vi "Digital Input DAQ Engine.vi"(8 "error in":errorcluster, 10 "DAQ Engine":refnum<notifier>, 11 "Sequence Context In":refnum<k7>) -> (0 "error out":errorcluster)   [LabVIEW 2023, in "LTT_TeststandSteptypes.lvlib"]
uses:
  LTT_TeststandSteptypes.lvlib
  HardwareAbstractionLayer_LVOOP/Main/Class Ref.ctl
  HardwareAbstractionLayer_LVOOP/DMM/DMM.lvclass
  HardwareAbstractionLayer_LVOOP/Function Generator/Function Generator.lvclass
  HardwareAbstractionLayer_LVOOP/Oscilloscope/Oscilloscope.lvclass
  HardwareAbstractionLayer_LVOOP/PowerSupply/PowerSupply.lvclass
  HardwareAbstractionLayer_LVOOP/Teststand/Teststand.lvclass
  HardwareAbstractionLayer_LVOOP/Analog Output/AO/AO.lvclass
  HardwareAbstractionLayer_LVOOP/Analog Input/AI/AI.lvclass
  HardwareAbstractionLayer_LVOOP/Database/Database.lvclass
  HardwareAbstractionLayer_LVOOP/Digital Output/DO_class/DO.lvclass
  HardwareAbstractionLayer_LVOOP/Digital Input/DI_class/DI.lvclass
  HardwareAbstractionLayer_LVOOP/PWM Output/PWM Output_class/PWM Output.lvclass
  HardwareAbstractionLayer_LVOOP/PWM Input/PWM Input_class/PWM Input.lvclass
  HardwareAbstractionLayer_LVOOP/NI Switch/NISwitch_class/NISwitch.lvclass
  HardwareAbstractionLayer_LVOOP/Modbus/Modbus_class/Modbus.lvclass
  HardwareAbstractionLayer_LVOOP/CAN/CAN Lib/CAN_class/CAN.lvclass
  HardwareAbstractionLayer_LVOOP/Digital Input/NI Digital Input_class/NI Digital Input.lvclass
  D:/eDCU LTT/VT LTT Project/Source Code/HardwareAbstractionLayer_LVOOP/Digital Input/DI_class/DI.lvclass
  HardwareAbstractionLayer_LVOOP/Main/Class Options.ctl
  <vilib>/Utility/error.llb/DialogType.ctl
  HardwareAbstractionLayer_LVOOP/Main/Main.lvclass
panel:
  in  "stop":bool
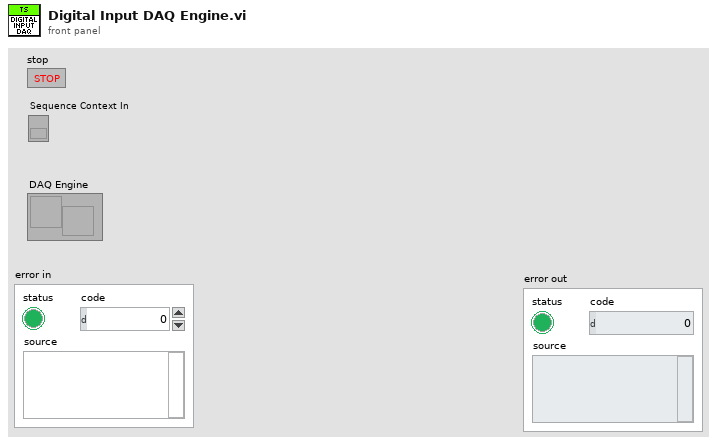
[diagram p1: front panel]
types:
  T1 = typedef "HardwareAbstractionLayer_LVOOP.lvlib/Main.lvclass/Class Ref.ctl" = cluster{"DMM":refnum<class "DMM.lvclass">, "Function Generator":refnum<class "Function Generator.lvclass">, "Oscilloscope":refnum<class "Oscilloscope.lvclass">, "PowerSupply":refnum<class "PowerSupply.lvclass">, "Teststand":refnum<class "Teststand.lvclass">, "AO":refnum<class "AO.lvclass">, "AI":refnum<class "AI.lvclass">, "Database":refnum<class "Database.lvclass">, "AO Waveform Generation":refnum<class "AO.lvclass">, "DO":refnum<class "DO.lvclass">, "DI":refnum<class "DI.lvclass">, "PWM Output":refnum<class "PWM Output.lvclass">, "PWM Input":refnum<class "PWM Input.lvclass">, "RelayOutput":refnum<class "NISwitch.lvclass">, "Modbus":refnum<class "Modbus.lvclass">, "CAN":refnum<class "CAN.lvclass">}
  T2 = typedef "HardwareAbstractionLayer_LVOOP.lvlib/Main.lvclass/Class Options.ctl" = enum16{"Init All Class", "Read All Class", "Write AI Class", "Write AO Class", "Write AO Waveform Generation", "Write DI Class", "Write DO Class", "Write PWM Input Class", "Write PWM Output Class", "Exit"}
  T3 = typedef "DialogType.ctl" = u16
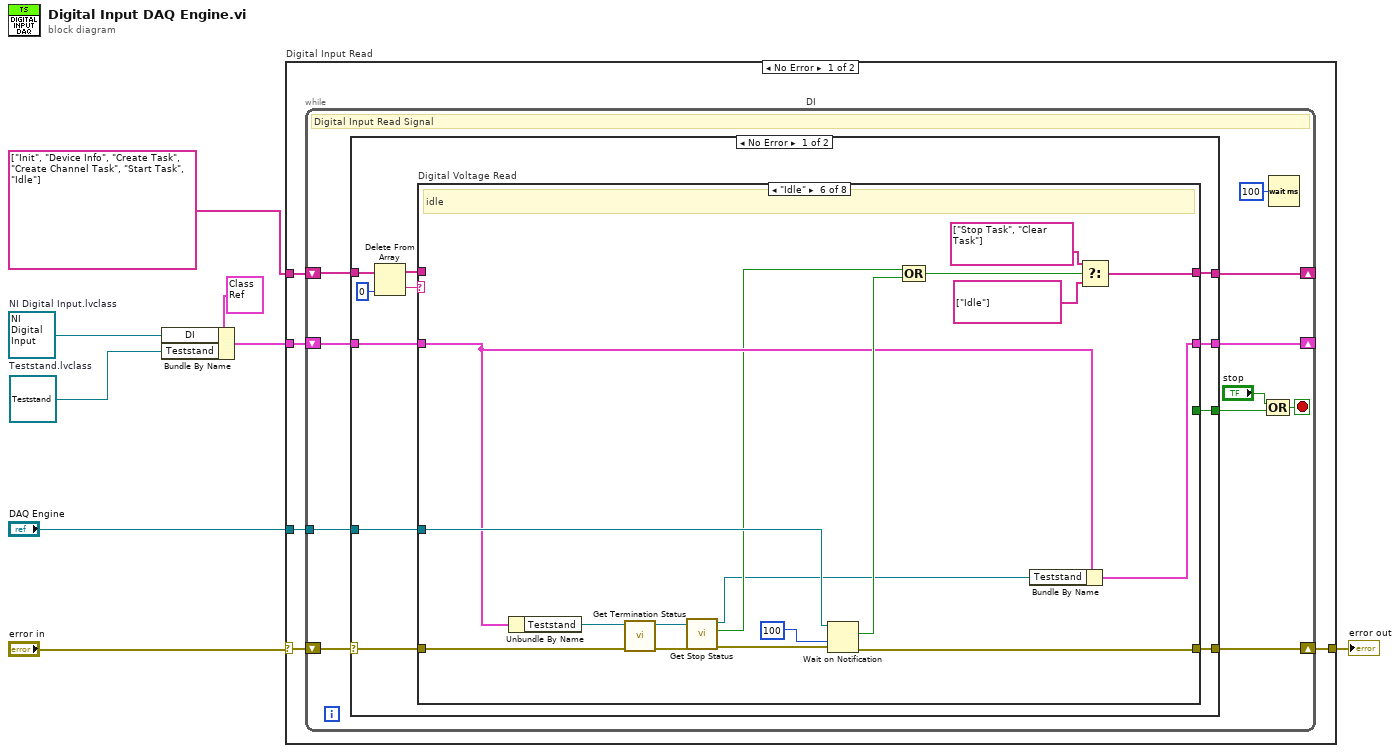
[diagram p0: block diagram]
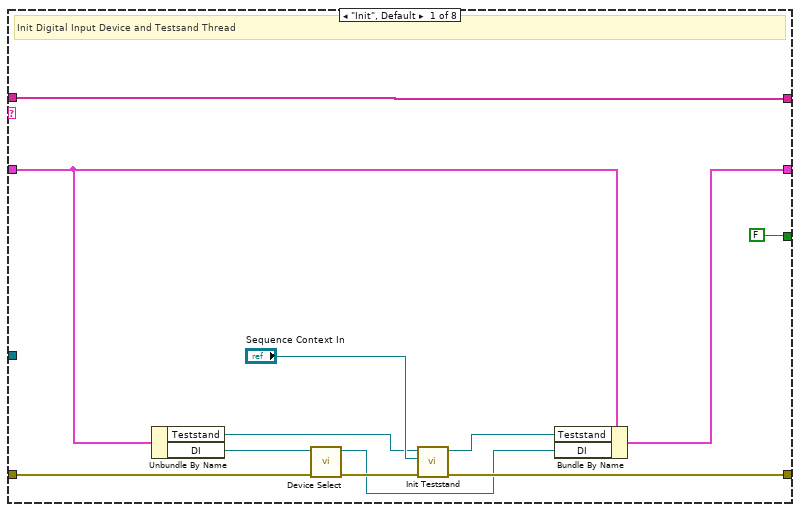
[diagram p2: hidden frame]
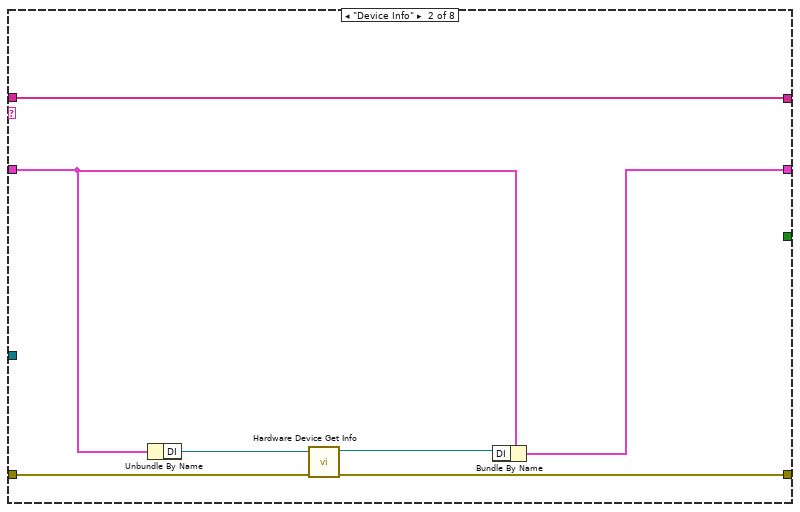
[diagram p3: hidden frame]
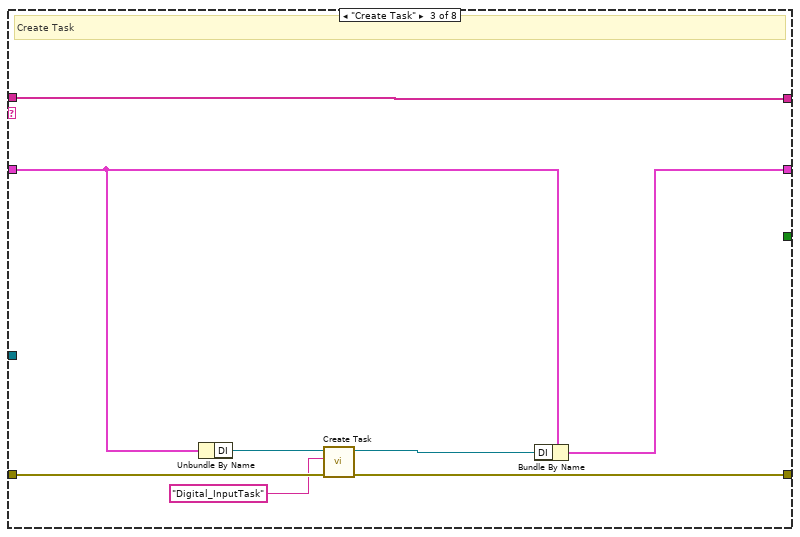
[diagram p4: hidden frame]
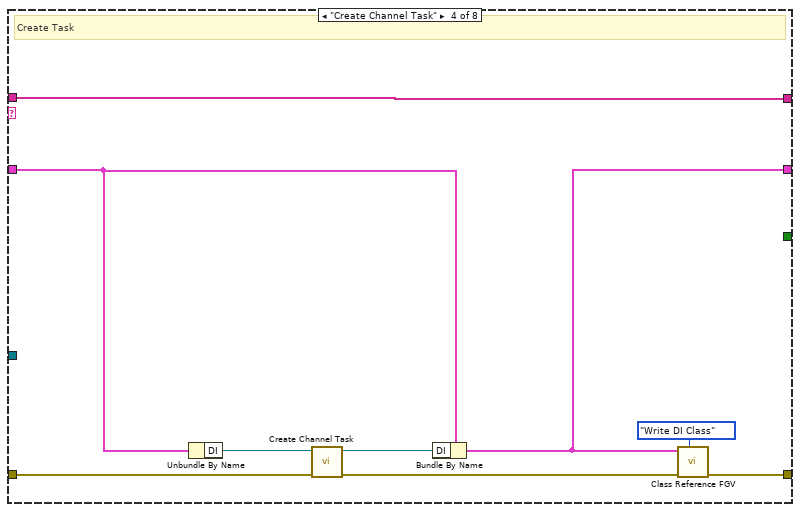
[diagram p5: hidden frame]
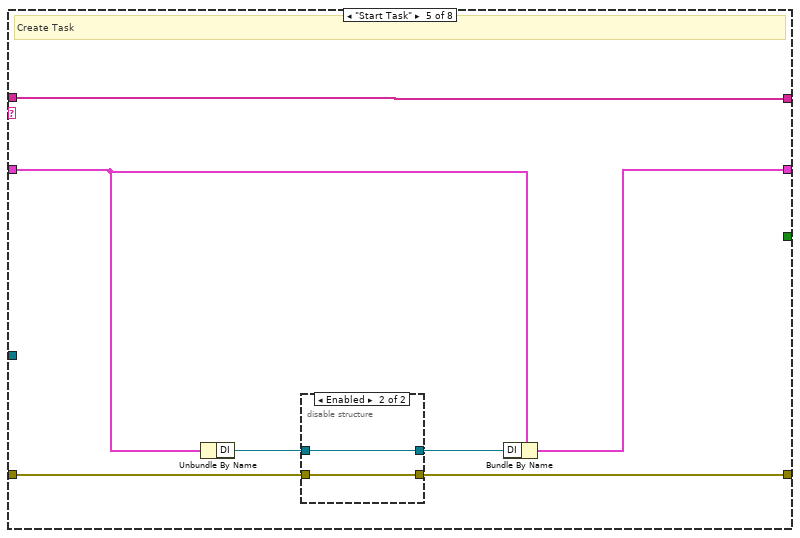
[diagram p6: hidden frame]
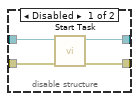
[diagram p7: hidden frame]
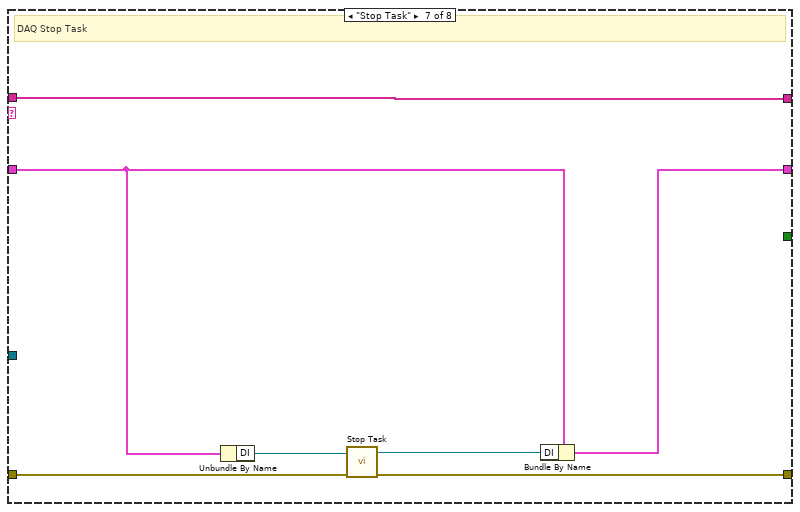
[diagram p8: hidden frame]
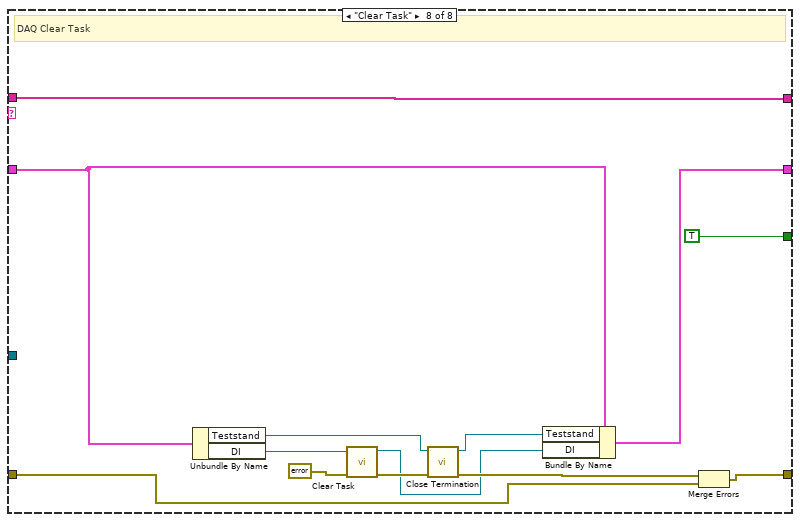
[diagram p9: hidden frame]
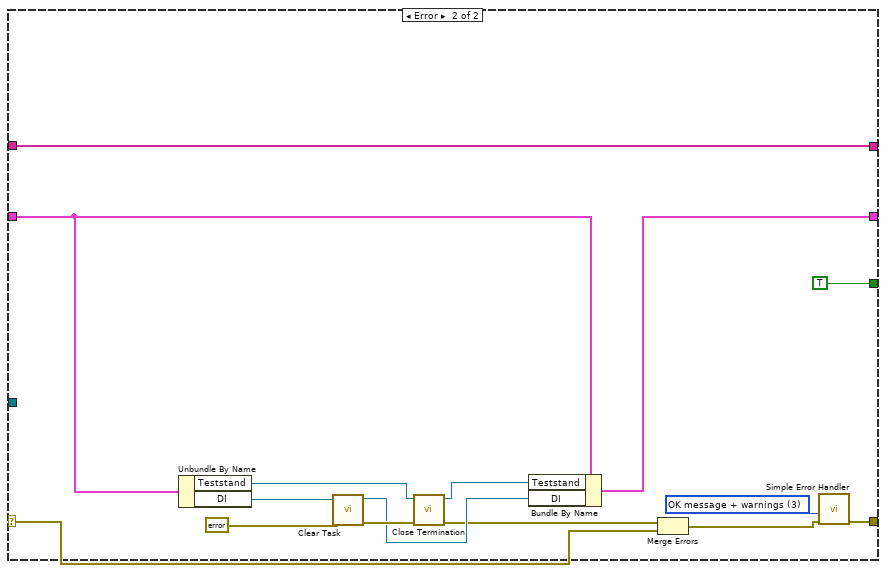
[diagram p10: hidden frame]
diagram:
  w1 = refnum<class "Teststand.lvclass"> refnum  # Teststand.lvclass
  w2 = refnum<class "NI Digital Input.lvclass"> refnum  # NI Digital Input.lvclass
  n1 = Bundle By Name(cluster=T1 {"DMM"=refnum, "Function Generator"=refnum, "Oscilloscope"=refnum, "PowerSupply"=refnum, "Teststand"=refnum, "AO"=refnum, "AI"=refnum, "Database"=refnum, "AO Waveform Generation"=refnum, "DO"=refnum, "DI"=refnum, "PWM Output"=refnum, "PWM Input"=refnum, "RelayOutput"=refnum, "Modbus"=refnum, "CAN"=refnum} ("Class Cluster"), "DI"=w2, "Teststand"=w1) -> (w5:T1)
  n2 = case "Digital Input Read" shown="No Error" "error in" {
    selector: "error in" -> [w13 w137]
    tunnel: [w12 w137] -> w7
    tunnel: w5 -> [w11 _]
    tunnel: string[] ["Init", "Device Info", "Create Task", "Create Channel Task", "Start Task", "Idle"] -> [w10 _]
    tunnel: "DAQ Engine" -> [w9 _]
    frame No Error {
      n3 = while "DI" {
        shift-right: [w23] -> w12
        shift-left: w13 -> [w24]
        shift-right: [w21] -> _
        shift-left: w11 -> [w22]
        shift-right: [w19] -> _
        shift-left: w10 -> [w20]
        tunnel: w9 -> [w14]
        stop <- w16 stop-if-true
        # "Digital Input Read Signal"
        n4 = case shown="No Error" w24 {
          selector: w24 -> [w35 w126]
          tunnel: [w34 w123] -> w23
          tunnel: w22 -> [w30 w129]
          tunnel: [w29 w127] -> w21
          tunnel: w20 -> [w33 w136]
          tunnel: [w27 w136] -> w19
          tunnel: [w26 TRUE] -> w15
          tunnel: w14 -> [w25 _]
          frame No Error {
            n5 = Delete From Array(array=w33, index=0) -> (deleted portion=w32:string, array with subset deleted=w28:string[])  [unwired: 1 in]
            n6 = case "Digital Voltage Read" shown="\"Idle\"" w32 {
              tunnel: w35 -> [w44 w52 w57 w69 w75 w91 w105 w109]
              tunnel: [w37 w51 w56 w65 w74 w96 w104 w111] -> w34
              tunnel: w30 -> [w46 w50 w61 w70 w77 w93 w107 w120]
              tunnel: [w45 w49 w60 w64 w76 w92 w106 w119] -> w29
              tunnel: w28 -> [w47 w54 w62 w71 w78 _ w108 w121]
              tunnel: [w47 w54 w62 w71 w78 w99 w108 w121] -> w27
              tunnel: [FALSE _ _ _ _ _ _ TRUE] -> w26
              tunnel: w25 -> [_ _ _ _ _ w97 _ _]
              frame "Init", Default {
                # "Init Digital Input Device and Testsand Thread"
                n7 = Unbundle By Name(w46) -> ("Teststand"=w40:refnum<class "Teststand.lvclass">, "DI"=w42:refnum<class "DI.lvclass">)
                n8 = call-dynamic "Device Select.vi"("error in (no error)"=w44, "DI in"=w42) -> ("error out"=w38:errorcluster, "DI out"=w36:refnum<class "DI.lvclass">)  [unwired: 8 in]
                n9 = call-dynamic "Init Teststand.vi"("error in (no error)"=w38, "Sequence Context In"="Sequence Context In", "Teststand in"=w40) -> ("error out"=w37:errorcluster, "Teststand out"=w39:refnum<class "Teststand.lvclass">)  [unwired: 7 in]
                n10 = Bundle By Name(cluster=w46, "Teststand"=w39, "DI"=w36) -> (w45:T1)
              }
              frame "Device Info" {
                n11 = Unbundle By Name(w50) -> ("DI"=w53:refnum<class "DI.lvclass">)
                n12 = call-dynamic "Hardware Device Get Info.vi"("error in (no error)"=w52, "DI in"=w53) -> ("error out"=w51:errorcluster, "DI out"=w48:refnum<class "DI.lvclass">)  [unwired: 8 in]
                n13 = Bundle By Name(cluster=w50, "DI"=w48) -> (w49:T1)
              }
              frame "Create Task" {
                # "Create Task"
                n14 = Unbundle By Name(w61) -> ("DI"=w59:refnum<class "DI.lvclass">)
                n15 = call-dynamic "Create Task.vi"("error in (no error)"=w57, "Task name"="Digital_InputTask", "DI in"=w59) -> ("error out"=w56:errorcluster, "DI out"=w58:refnum<class "DI.lvclass">)  [unwired: 7 in]
                n16 = Bundle By Name(cluster=w61, "DI"=w58) -> (w60:T1)
              }
              frame "Create Channel Task" {
                # "Create Task"
                n17 = Unbundle By Name(w70) -> ("DI"=w68:refnum<class "DI.lvclass">)
                n18 = call-dynamic "Create Channel Task.vi"("error in (no error)"=w69, "DI in"=w68) -> ("error out"=w66:errorcluster, "DI out"=w67:refnum<class "DI.lvclass">)  [unwired: 8 in]
                n19 = Bundle By Name(cluster=w70, "DI"=w67) -> (w64:T1)
                n20 = call "Class Reference FGV.vi"("Options"=Class_Options."Write DI Class", "error in"=w66, "Class Cluster In"=w64) -> ("error out"=w65:errorcluster)  [unwired: 7 in, 1 out]
              }
              frame "Start Task" {
                # "Create Task"
                n21 = Unbundle By Name(w77) -> ("DI"=w73:refnum<class "DI.lvclass">)
                n22 = disable-structure shown="Enabled" {
                  disable-tunnel: w75 -> [w82 w84]
                  disable-tunnel: [w81 w84] -> w74
                  disable-tunnel: w73 -> [w80 w83]
                  disable-tunnel: [w79 w83] -> w72
                  frame Disabled {
                    n23 = call-dynamic "Start Task.vi"("error in (no error)"=w82, "DI in"=w80) -> ("error out"=w81:errorcluster, "DI out"=w79:refnum<class "DI.lvclass">)  [unwired: 8 in]
                  }
                  frame Enabled {
                  }
                }
                n24 = Bundle By Name(cluster=w77, "DI"=w72) -> (w76:T1)
              }
              frame "Idle" {
                # "idle"
                n25 = Unbundle By Name(w93) -> ("Teststand"=w90:refnum<class "Teststand.lvclass">)
                n26 = call-dynamic "Get Termination Status.vi"("error in (no error)"=w91, "Teststand in"=w90) -> ("error out"=w89:errorcluster, "Teststand out"=w87:refnum<class "Teststand.lvclass">)  [unwired: 7 in, 1 out]
                n27 = call-dynamic "Get Stop Status.vi"("error in (no error)"=w89, "Teststand in"=w87) -> ("error out"=w88:errorcluster, "Value"=w86:bool, "Teststand out"=w85:refnum<class "Teststand.lvclass">)  [unwired: 7 in]
                n28 = Wait on Notification(notifier=w97, timeout in ms (-1)=100, error in (no error)=w88) -> (notification=w94:bool, error out=w96:errorcluster)  [unwired: 1 in, 2 out]
                n29 = Compound Arithmetic op=OR(w86, w94) -> (w98:bool)
                n30 = Bundle By Name(cluster=w93, "Teststand"=w85) -> (w92:T1)
                n31 = Select(t=string[] ["Stop Task", "Clear Task"], s=w98, f=string[] ["Idle"]) -> (s? t:f=w99:string[])
              }
              frame "Stop Task" {
                # "DAQ Stop Task"
                n32 = Unbundle By Name(w107) -> ("DI"=w103:refnum<class "DI.lvclass">)
                n33 = call-dynamic "Stop Task.vi"("error in (no error)"=w105, "DI in"=w103) -> ("error out"=w104:errorcluster, "DI out"=w102:refnum<class "DI.lvclass">)  [unwired: 8 in]
                n34 = Bundle By Name(cluster=w107, "DI"=w102) -> (w106:T1)
              }
              frame "Clear Task" {
                # "DAQ Clear Task"
                n35 = Unbundle By Name(w120) -> ("Teststand"=w116:refnum<class "Teststand.lvclass">, "DI"=w118:refnum<class "DI.lvclass">)
                n36 = call-dynamic "Clear Task.vi"("error in (no error)"=errorcluster {"status"=FALSE, "code"=0, "source"=""}, "DI in"=w118) -> ("error out"=w114:errorcluster, "DI out"=w112:refnum<class "DI.lvclass">)  [unwired: 8 in]
                n37 = call-dynamic "Close Termination.vi"("error in (no error)"=w114, "Teststand in"=w116) -> ("error out"=w113:errorcluster, "Teststand out"=w115:refnum<class "Teststand.lvclass">)  [unwired: 8 in]
                n38 = Bundle By Name(cluster=w120, "Teststand"=w115, "DI"=w112) -> (w119:T1)
                n39 = Merge Errors(w113, w109) -> (w111:errorcluster)
              }
            }
          }
          frame Error {
            w122 = T3 3 items=["no dialog", "OK message", "continue or stop message", "OK message + warnings", "continue/stop + warnings"] ("type of dialog (OK msg:1)")
            n40 = Unbundle By Name(w129) -> ("Teststand"=w133:refnum<class "Teststand.lvclass">, "DI"=w134:refnum<class "DI.lvclass">)
            n41 = call-dynamic "Clear Task.vi"("error in (no error)"=errorcluster {"status"=FALSE, "code"=0, "source"=""}, "DI in"=w134) -> ("error out"=w131:errorcluster, "DI out"=w130:refnum<class "DI.lvclass">)  [unwired: 8 in]
            n42 = call-dynamic "Close Termination.vi"("error in (no error)"=w131, "Teststand in"=w133) -> ("error out"=w128:errorcluster, "Teststand out"=w132:refnum<class "Teststand.lvclass">)  [unwired: 8 in]
            n43 = Bundle By Name(cluster=w129, "Teststand"=w132, "DI"=w130) -> (w127:T1)
            n44 = Merge Errors(w128, w126) -> (w124:errorcluster)
            n45 = call <vilib>:"Simple Error Handler.vi"("type of dialog (OK msg:1)"=w122, "error in (no error)"=w124) -> ("error out"=w123:errorcluster)  [unwired: 3 in, 4 out]
          }
        }
        n46 = Compound Arithmetic op=OR("stop", w15) -> (w16:bool)
        n47 = Wait (ms)(milliseconds to wait=u32 100) -> ()  [unwired: 1 out]
      }
    }
    frame Error {
      # "Error"
    }
  }
  "error out" <- w7
